vi "Scan_Hopping_CV.vi"() -> ()   [LabVIEW 2023]
uses:
  Sub_Vi/TypeDefs/Settings.ctl
  Sub_Vi/TypeDefs/ChangeOnFly.ctl
  Sub_Vi/TypeDefs/Display.ctl
  Settings.vi
panel:
  in  "NumberOfCVsAtEachPoint":i32=1
  in  "Hopping Distance Between Lines (um)":dbl=1.0
  in  "Pre CV HoldTime /s":dbl=10.0 format="%#_13g"
  in  "CV Rate / V/s":dbl=0.2
  in  "Voltage to Electrode (V) 3":dbl=-2.0
  in  "Voltage to Electrode (V) 2":dbl=1.0
  out "Estimated Time (mins)":dbl
  in  "Display Cluster":T1
  in  "ChangeonFly":T2
  in  "SettingsCluster":T3={"Sample Rate (us)"=1, "Samples Per Data Point (int, power of 2)"=1000, "DistanceToBulk (um)"=-1.0, "HoldTimeScaler"=40000, "SaveData"=TRUE, "DistanceToBulk (um) 2"=-1.0, "DistanceToBulk (um) 3"=-1.0}
  in  "Retract after approach over (T/F)":bool=TRUE
  in  "Feedback Type":T4(ring)=enum."Current 1"
  in  "StopCond_GreaterThan?":bool
  in  "Approach Rate Hopping (um/s)":dbl=0.15
  in  "Retract Rate (um/s)":dbl=1.0
  in  "Hopping Distance Along Line(um)":dbl=1.0
  in  "Z End (um)":dbl=38.0
  in  "Distance To Retract (um)":dbl=-5.0
  in  "Upper dZ limit":i32=8
  in  "Feedback Threshold\nAbsolute value":dbl=-1e-09
  in  "P":fxp<+/-,32,1>=0.029999999795109034 format="%.32g"
  in  "X Center (um)":dbl=150.0 min=0.0 max=300.0
  in  "Y Center (um)":dbl=150.0 min=0.0 max=300.0
  in  "Y Width (um)":dbl=10.0
  in  "X Width (um)":dbl=10.0
  in  "Scan Rate (um/s)":dbl=5.0
  in  "Voltage to Electrode (V)":dbl=-0.4
  in  "Approach Rate (um/s)":dbl=0.2
  in  "Z Start height (um)":dbl
  in  "Start scan Button":bool
  in  "Stop":bool
  in  "Pause":bool
  in  "Start Scanning Button":bool
  out "Y end":dbl
  out "X end":dbl
  out "X start":dbl
  out "Y start":dbl
  in  "Tab Control 4":T5(tab)=enum."Current Follower 3"
  out "Topology":dbl[][](graph)
  out "Current 1":dbl[][](graph)
  out "Current 2":dbl[][](graph)
  out "Current 3":dbl[][](graph)
  out "V vs C1":cluster{"Y":dbl[], "Y":dbl[]}[](graph)
  out "Z vs C3":cluster{"Y":dbl[], "Y":dbl[]}[](graph)
  out "Lock in Phase":dbl[](graph)
  out "Lock in amp":dbl[](graph)
  out "t vs C1":dbl[](graph)
  out "Z vs C1":cluster{"Y":dbl[], "Y":dbl[]}[](graph)
  # "Feedback  Settings"
  # "Approach  Settings"
  # "Scan  Settings"
  # "Advanced Settings"
  # "Define Scan area \nAbout centre"
  # "Change top/bottom values \ndepending on scan"
  # "Change top/bottom values \ndepending on scan"
  # "Change top/bottom values \ndepending on scan"
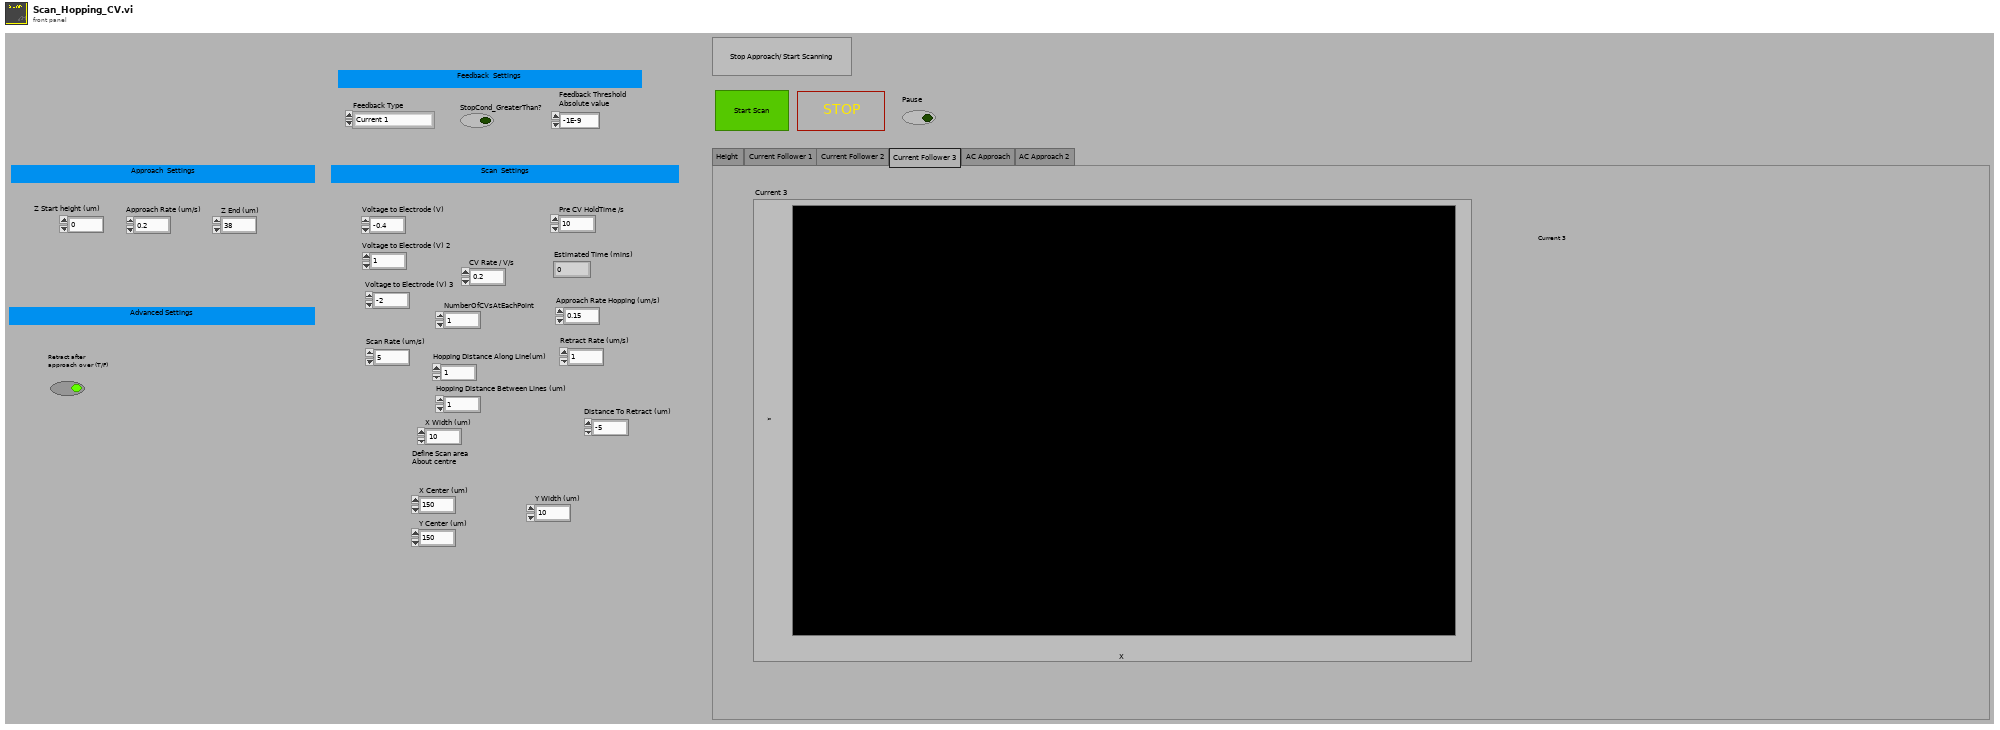
[diagram p1: front panel]
types:
  T1 = typedef "Display.ctl" = cluster{"X":refnum<vi>, "Y":refnum<vi>, "Z":refnum<vi>, "Amp":refnum<vi>, "Phase":refnum<vi>, "t vs Z":refnum<vi>, "t vs C1":refnum<vi>, "t vs C2":refnum<vi>, "t vs C3":refnum<vi>, "t vs Amp":refnum<vi>, "t vs Phase":refnum<vi>, "t vs X":refnum<vi>, "t vs Y":refnum<vi>, "Z vs C1":refnum<vi>, "Z vs C2":refnum<vi>, "Z vs C3":refnum<vi>, "V vs C1":refnum<vi>, "V vs C2":refnum<vi>, "V vs C3":refnum<vi>, "X/Y/Z F":refnum<vi>, "X/Y/Z R":refnum<vi>, "X/Y/C1 F":refnum<vi>, "X/Y/C1 R":refnum<vi>, "X/Y/C2 F":refnum<vi>, "X/Y/C2 R":refnum<vi>, "X/Y/C3 F":refnum<vi>, "X/Y/C3 R":refnum<vi>, "NumberOfLines":u16, "um Per Pixel":dbl, "um Per Line":dbl, "X Center":dbl, "Hop X/Y/Z":refnum<vi>, "Hop X/Y/C1":refnum<vi>, "Hop X/Y/C2":refnum<vi>, "Hop X/Y/C3":refnum<vi>, "X Width":dbl, "Y Width":dbl, "Hopping Distance":dbl, "V2 vs C1":refnum<vi>, "V vs Phase":refnum<vi>, "Y Center":dbl, "Number of Pixels":dbl, "V2 vs C2":refnum<vi>, "V2 vs C3":refnum<vi>, "V vs y":refnum<vi>, "V2 vs y":refnum<vi>, "Z vs Amp":refnum<vi>, "Z vs Phase":refnum<vi>}
  T2 = typedef "ChangeOnFly.ctl" = cluster{"Stop (boolean)":refnum<vi>, "Pause (boolean)":refnum<vi>, "EndCurrentLine (boolean)":refnum<vi>, "max movement per update step (Interger, nm)":refnum<vi>, "P (float, arb)":refnum<vi>, "Feedback set point (double, Amps)":refnum<vi>, "Voltage (double, V)":refnum<vi>, "Feedback set point 2 (double, Amps)":refnum<vi>, "Stop on Greater Than 2? (boolean)":refnum<vi>, "Stop on Greater Than? (boolean)":refnum<vi>, "Voltage 2 (double, V)":refnum<vi>, "Feedback Type (enum)":refnum<vi>, "Feedback Type 2 (enum)":refnum<vi>}
  T3 = typedef "Settings.ctl" = cluster{"Sample Rate (us)":u32, "Samples Per Data Point (int, power of 2)":i16, "DistanceToBulk (um)":dbl, "HoldTimeScaler":u64, "SaveData":bool, "DistanceToBulk (um) 2":dbl, "DistanceToBulk (um) 3":dbl}
  T4 = enum16{"AC Magnitude", "Current 1", "Current 2", "Phase"}
  T5 = enum32{"Height", "Current Follower 1", "Current Follower 2", "Current Follower 3", "AC Approach", "AC Approach 2"}
  T6 = cluster{"Scan Rate (um/s)":dbl, "X Start":dbl, "X End":dbl, "Y Start":dbl, "Y End":dbl, " Z Start":dbl, "HoppingDistance":dbl, "V":dbl, "Z End":dbl, "Approach Rate Hopping (um/s)":dbl, "Retrack Rate (um/s)":dbl, "V 2":dbl, "Approach Rate (um/s)":dbl, "V 3":dbl, "CV Rate / V/s":dbl, "V 4":dbl, "V 1":dbl, "HoldTime1/s":dbl, "Hold time 2 / s":dbl, "Hold time 3/ s":dbl, "HoppingDistanceBetweenLines":dbl}
  T7 = typedef "WayPointCluster.ctl" = cluster{"X (um)":dbl[], "Y (um)":dbl[], "Z (um)":dbl[], "V (V)":dbl[], "X Velocity (um s-1)":dbl[], "Y Velocity (um s-1)":dbl[], "Z Velocity (um s-1)":dbl[], "V Velocity (V s-1)":dbl[], "FeedBack Type (enum)":u16[], "Move X (boolean)":bool[], "Move Y (boolean)":bool[], "Move Z (boolean)":bool[], "Move V (boolean)":bool[], "Jump V (boolean)":bool[], "Hold (boolean)":bool[], "Hold Time":u32[], "V2 (V)":dbl[], "Move V2":bool[], "V2 Velocity (V s-1)":dbl[], "Jump V2 (boolean)":bool[], "Update z Position delta (ms)":i16[], "Hold Feedback1":bool[], "Move Z PicoMotor":bool[], " Z PicoMotor Direction":bool[], "DIO0":bool[]}
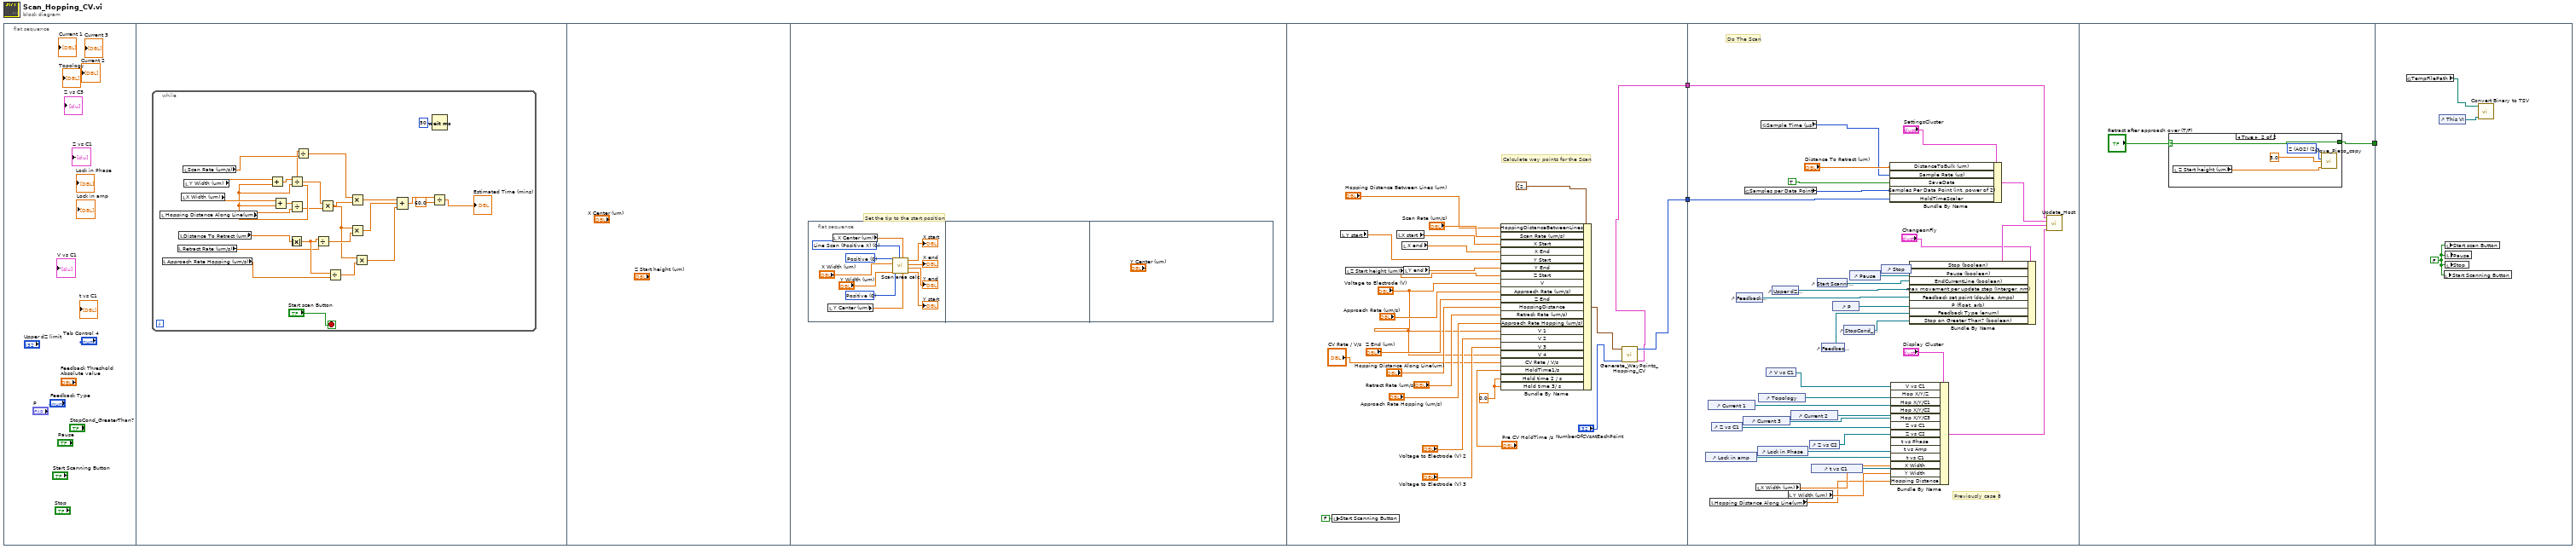
[diagram p0: block diagram]
diagram:
  n1 = flat-sequence {
    tunnel: [w41] -> w3
    tunnel: [w42] -> w1
    tunnel: w3 -> [w95]
    tunnel: w1 -> [w63]
    tunnel: [w96] -> w2
    tunnel: w2 -> [_]
    frame #0 {
    }
    frame #1 {
      n2 = while {
        stop <- "Start scan Button" stop-if-true
        n3 = local read "Hopping Distance Along Line(um)"() -> (w8:dbl)
        n4 = local read "Approach Rate Hopping (um/s)"() -> (w11:dbl)
        n5 = local read "Retract Rate (um/s)"() -> (w12:dbl)
        n6 = local read "Distance To Retract (um)"() -> (w13:dbl)
        n7 = local read "X Width (um)"() -> (w17:dbl)
        n8 = local read "Scan Rate (um/s)"() -> (w19:dbl)
        n9 = local read "Y Width (um)"() -> (w18:dbl)
        n10 = Add(x=w18, y=w8) -> (x+y=w10:dbl)
        n11 = Add(x=w17, y=w8) -> (x+y=w9:dbl)
        n12 = Absolute Value(x=w13) -> (abs(x)=w14:dbl)
        n13 = Divide(x=w10, y=w8) -> (x/y=w6:dbl)
        n14 = Divide(x=w9, y=w8) -> (x/y=w5:dbl)
        n15 = Divide(x=w8, y=w19) -> (x/y=w20:dbl)
        n16 = Divide(x=w14, y=w12) -> (x/y=w22:dbl)
        n17 = Multiply(x=w6, y=w5) -> (x*y=w7:dbl)
        n18 = Divide(x=w14, y=w11) -> (x/y=w15:dbl)
        n19 = Multiply(x=w20, y=w7) -> (x*y=w21:dbl)
        n20 = Multiply(x=w7, y=w22) -> (x*y=w23:dbl)
        n21 = Multiply(x=w7, y=w15) -> (x*y=w16:dbl)
        n22 = Compound Arithmetic op=ADD(w21, w23, w16) -> (w24:dbl)
        n23 = Divide(x=w24, y=60.0) -> (x/y=→"Estimated Time (mins)":dbl)
        n24 = Wait (ms)(milliseconds to wait=u32 50) -> ()  [unwired: 1 out]
      }
    }
    frame #2 {
    }
    frame #3 {
      # "Set the tip to the start position"
      n25 = flat-sequence {
        frame #0 {
          w28 = u16 0 items=["Positive", "Negative"] ("Major Axis Direction")
          w29 = u16 0 items=["Positive", "Negative"] ("Minor Axis Direction")
          w30 = u16 0 items=["Line Scan (Positive X)", "Line Scan (Negative X)", "Line Scan (Positive Y)", "Line Scan (Negative Y)"] ("Scan Type")
          n26 = local read "Y Center (um)"() -> (w31:dbl)
          n27 = local read "X Center (um)"() -> (w32:dbl)
          n28 = call "Scan area calc.vi"("Y Width"="Y Width (um)", "Major Axis Direction"=w28, "X Width"="X Width (um)", "Minor Axis Direction"=w29, "Scan Type"=w30, "Y Center"=w31, "X Center"=w32) -> ("Y start"=→"Y start":dbl, "Y end"=→"Y end":dbl, "X end"=→"X end":dbl, "X start"=→"X start":dbl)
        }
        frame #1 {
        }
        frame #2 {
        }
      }
    }
    frame #4 {
      w46 = 0.0 ("HoldTime1/s")
      # "Calculate way points for the Scan"
      n29 = local write "Start Scanning Button"(FALSE ("Start Scanning Button")) -> ()
      n30 = local read "Y start"() -> (w51:dbl)
      n31 = local read "Z Start height (um)"() -> (w56:dbl)
      n32 = local read "X start"() -> (w61:dbl)
      n33 = local read "X end"() -> (w60:dbl)
      n34 = local read "Y end"() -> (w59:dbl)
      n35 = Bundle By Name(cluster=T6 {"Scan Rate (um/s)"=20.0, "X Start"=180.0, "X End"=220.0, "Y Start"=199.0, "Y End"=201.0, " Z Start"=0.0, "HoppingDistance"=0.5, "V"=0.0, "Z End"=38.0, "Approach Rate Hopping (um/s)"=0.5, "Retrack Rate (um/s)"=20.0, "V 2"=0.0, "Approach Rate (um/s)"=0.5, "V 3"=0.0, "CV Rate / V/s"=1.0, "V 4"=0.0, "V 1"=0.0, "HoldTime1/s"=0.5, "Hold time 2 / s"=0.0, "Hold time 3/ s"=0.0, "HoppingDistanceBetweenLines"=0.5} ("Input Cluster"), "HoppingDistanceBetweenLines"="Hopping Distance Between Lines (um)", "Scan Rate (um/s)"="Scan Rate (um/s)", "X Start"=w61, "X End"=w60, "Y Start"=w51, "Y End"=w59, "Z Start"=w56, "V"="Voltage to Electrode (V)", "Approach Rate (um/s)"="Approach Rate (um/s)", "Z End"="Z End (um)", "HoppingDistance"="Hopping Distance Along Line(um)", "Retrack Rate (um/s)"="Retract Rate (um/s)", "Approach Rate Hopping (um/s)"="Approach Rate Hopping (um/s)", "V 1"="Voltage to Electrode (V)", "V 2"="Voltage to Electrode (V) 2", "V 3"="Voltage to Electrode (V) 3", "V 4"="Voltage to Electrode (V)", "CV Rate / V/s"="CV Rate / V/s", "HoldTime1/s"="Pre CV HoldTime /s", "Hold time 2 / s"=w46, "Hold time 3/ s"=w46) -> (w40:T6)
      n36 = call "Generate_WayPoints_Hopping_CV.vi"("NumberOfCVsAtEachPoint"="NumberOfCVsAtEachPoint", "Input Cluster"=w40) -> ("output cluster"=w41:T7, "WaitTimeScaler"=w42:u64)  [unwired: 8 in]
    }
    frame #5 {
      # "Previously case 8"
      # "Do The Scan"
      n37 = control-ref of="Lock in amp"() -> (w84:refnum<vi>)
      n38 = control-ref of="Current 1"() -> (w78:refnum<vi>)
      n39 = local read "Hopping Distance Along Line(um)"() -> (w74:dbl)
      n40 = control-ref of="Z vs C1"() -> (w81:refnum<vi>)
      n41 = control-ref of="Feedback Threshold\nAbsolute value"() -> (w88:refnum<vi>)
      n42 = control-ref of="Current 3"() -> (w80:refnum<vi>)
      n43 = global read "Settings.vi" "Samples per Data Point"() -> (w70:u16)
      n44 = local read "X Width (um)"() -> (w76:dbl)
      n45 = control-ref of="Lock in Phase"() -> (w83:refnum<vi>)
      n46 = control-ref of="Topology"() -> (w77:refnum<vi>)
      n47 = global read "Settings.vi" "Sample Time (µs)"() -> (w65:u32)
      n48 = control-ref of="V vs C1"() -> (w66:refnum<vi>)
      n49 = control-ref of="Upper dZ limit"() -> (w90:refnum<vi>)
      n50 = local read "Y Width (um)"() -> (w75:dbl)
      n51 = control-ref of="Current 2"() -> (w79:refnum<vi>)
      n52 = control-ref of="Z vs C2"() -> (w82:refnum<vi>)
      n53 = control-ref of="t vs C1"() -> (w85:refnum<vi>)
      n54 = control-ref of="Start Scanning Button"() -> (w91:refnum<vi>)
      n55 = control-ref of="Feedback Type"() -> (w68:refnum<vi>)
      n56 = control-ref of="P"() -> (w89:refnum<vi>)
      n57 = control-ref of="StopCond_GreaterThan?"() -> (w69:refnum<vi>)
      n58 = control-ref of="Pause"() -> (w87:refnum<vi>)
      n59 = control-ref of="Stop"() -> (w86:refnum<vi>)
      n60 = Bundle By Name(cluster="SettingsCluster", "DistanceToBulk (um)"="Distance To Retract (um)", "Sample Rate (us)"=w65, "SaveData"=TRUE ("Save Data"), "Samples Per Data Point (int, power of 2)"=w70, "HoldTimeScaler"=w63) -> (w93:T3)
      n61 = Bundle By Name(cluster="Display Cluster", "V vs C1"=w66, "Hop X/Y/Z"=w77, "Hop X/Y/C1"=w78, "Hop X/Y/C2"=w79, "Hop X/Y/C3"=w80, "Z vs C1"=w81, "Z vs C2"=w82, "t vs Phase"=w83, "t vs Amp"=w84, "t vs C1"=w85, "X Width"=w76, "Y Width"=w75, "Hopping Distance"=w74) -> (w94:T1)
      n62 = Bundle By Name(cluster="ChangeonFly", "Stop (boolean)"=w86, "Pause (boolean)"=w87, "EndCurrentLine (boolean)"=w91, "max movement per update step (Interger, nm)"=w90, "Feedback set point (double, Amps)"=w88, "P (float, arb)"=w89, "Feedback Type (enum)"=w68, "Stop on Greater Than? (boolean)"=w69) -> (w92:T2)
      n63 = call "Update_Host.vi"("Display Cluster"=w94, "ChangeonFly"=w92, "SettingsCluster"=w93, "WayPointCluster"=w95) -> ()  [unwired: 6 in]
    }
    frame #6 {
      n64 = case shown="True" "Retract after approach over (T/F)" {
        selector: "Retract after approach over (T/F)" -> [w98 w99]
        tunnel: [w98 w99] -> w96
        frame False {
        }
        frame True {
          w102 = u16 2 items=["X (AO0)", "Y (AO1)", "Z (AO2)", "V (AO3)"] ("Channel")
          n65 = local read "Z Start height (um)"() -> (w100:dbl)
          n66 = call "Move_Piezo_copy.vi"("Piezo"=w102, "Movement Speed (µm/s)"=5.0 ("Scan Rate (um/s)"), "Position (µm) (or V)"=w100) -> ()  [unwired: 13 in]
        }
      }
    }
    frame #7 {
      w105 = FALSE ("Stop")
      n67 = global read "Settings.vi" "TempFilePath"() -> (w103:path)
      n68 = control-ref of="This VI"() -> (w104:refnum<vi>)
      n69 = local write "Start Scanning Button"(w105) -> ()
      n70 = local write "Start scan Button"(w105) -> ()
      n71 = local write "Pause"(w105) -> ()
      n72 = local write "Stop"(w105) -> ()
      n73 = call "Convert Binary to TSV.vi"("This VI"=w104, "TDMS DataFile Name"=w103) -> ()  [unwired: 10 in]
    }
  }
